vi "NS Length.vi"(10 "m-nm NS base":dbl caption="m-nm 4", 11 "Length of Base":dbl) -> (3 "Numeric":dbl)   [LabVIEW 2020]
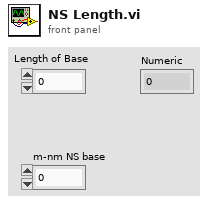
[diagram p1: front panel]
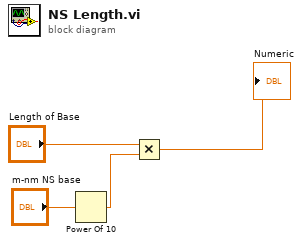
[diagram p0: block diagram]
diagram:
  n1 = Power Of 10(x="m-nm NS base") -> (10^x=w2:dbl)
  n2 = Multiply(x="Length of Base", y=w2) -> (x*y=→"Numeric":dbl)
